vi "File Namer.vi"() -> ()   [LabVIEW 2024]
uses:
  Controls/MainStates.ctl
  <userlib>/_OpenG.lib/array/array.llb/Remove Duplicates from 1D Array (String)__ogtk.vi
  <userlib>/_OpenG.lib/array/array.llb/openg_array.lvlib
panel:
  in  "Clean after \"(\"":bool
  out "New":string
  out "Old":string
  out "new path":path
  in  "Auto":enum32{"Manual", "MKV", "AVI", "MP4", "MP3"}(radio)
  in  "Commit":bool
  in  "Replacement String":string
  in  "Split Key":string="("
  in  "Method":T1(ring)
  in  "Extension":string=".*"
  in  "Path":path
  out "New":i32(listbox)
  out "Current":i32(listbox)=1
  in  "Exit":bool
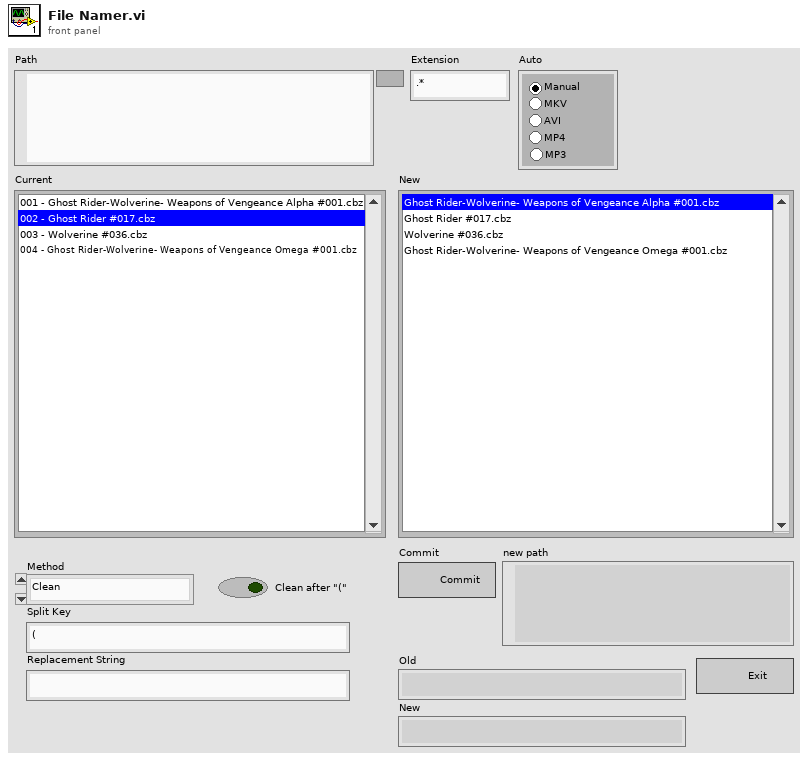
[diagram p1: front panel]
types:
  T1 = enum16{"Clean", "Replace", "Clear Periods", "Strip Prefix", "Add Prefix"}
  T2 = typedef "MainStates.ctl" = enum16{"Init", "Get Path", "Get Files", "Set Extension", "Check for Dups", "Clean", "Add Prefix", "Replace", "Periods", "Strip Prefix", "Commit", "Wait for Input", "Exit"}
  T3 = enum8{"Enabled", "Disabled", "Disabled and Grayed Out"}
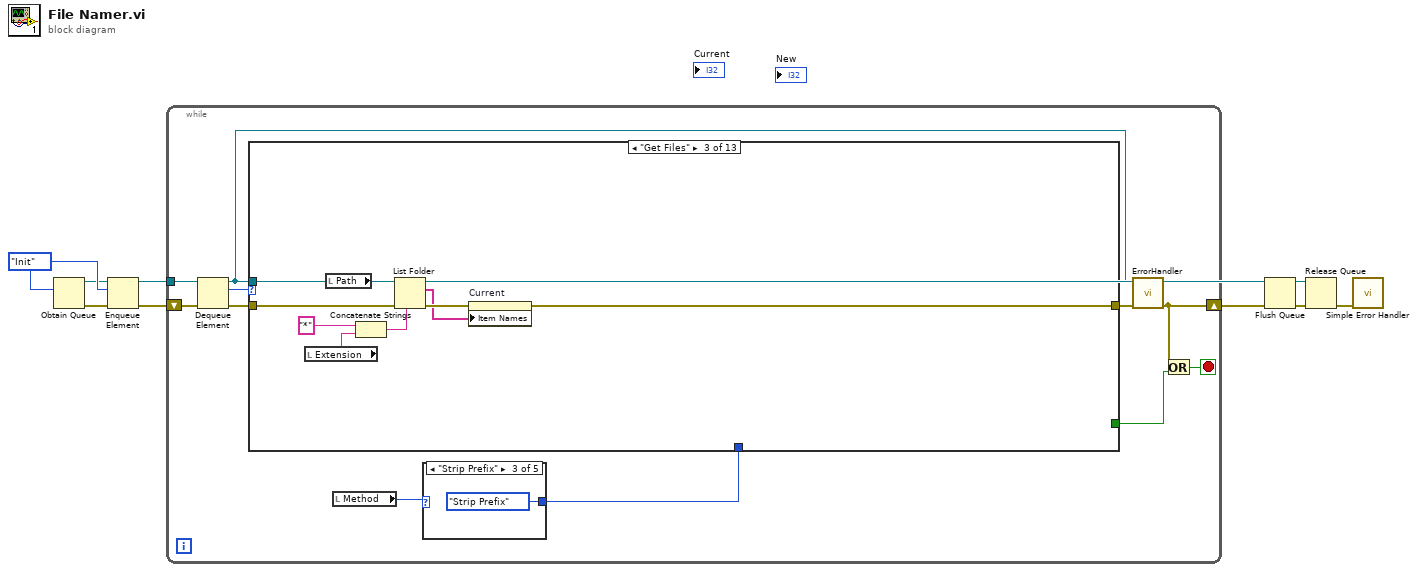
[diagram p0: block diagram]
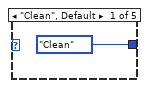
[diagram p2: hidden frame]
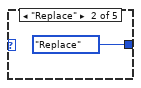
[diagram p3: hidden frame]
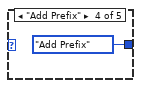
[diagram p4: hidden frame]
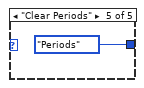
[diagram p5: hidden frame]
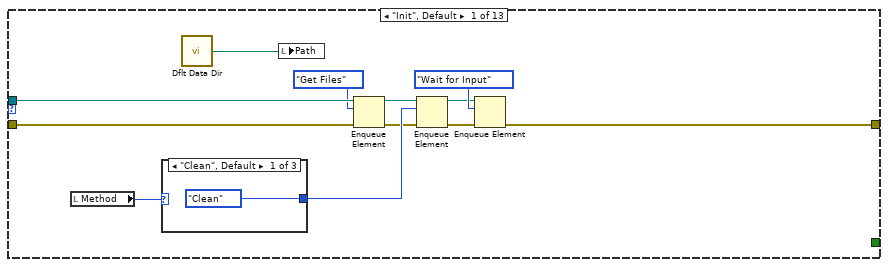
[diagram p6: hidden frame]
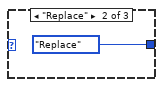
[diagram p7: hidden frame]
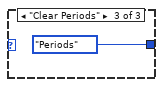
[diagram p8: hidden frame]
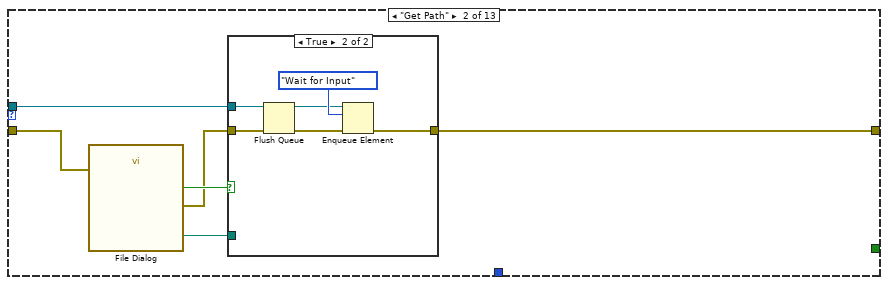
[diagram p9: hidden frame]
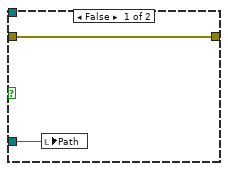
[diagram p10: hidden frame]
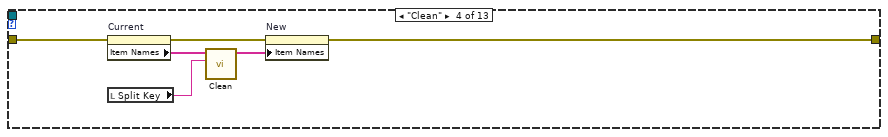
[diagram p11: hidden frame]
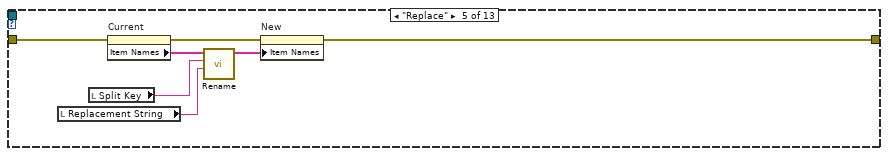
[diagram p12: hidden frame]
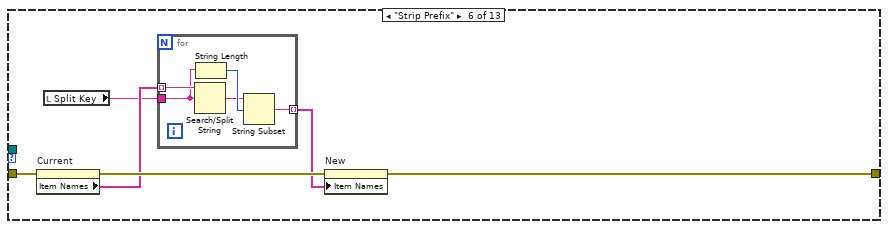
[diagram p13: hidden frame]
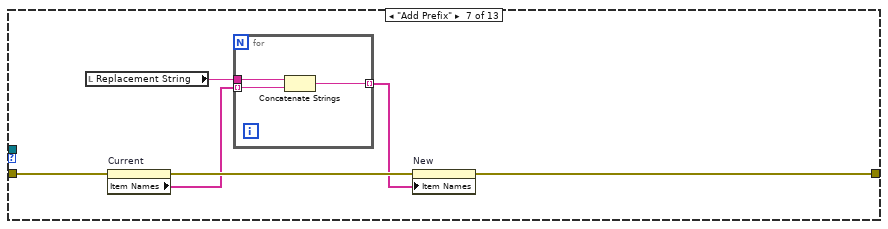
[diagram p14: hidden frame]
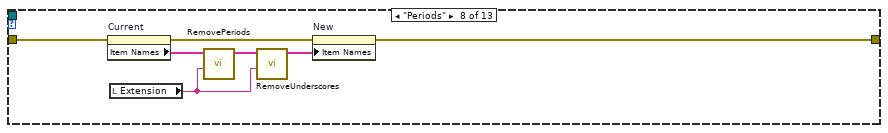
[diagram p15: hidden frame]
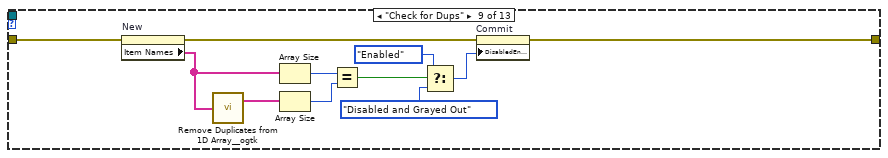
[diagram p16: hidden frame]
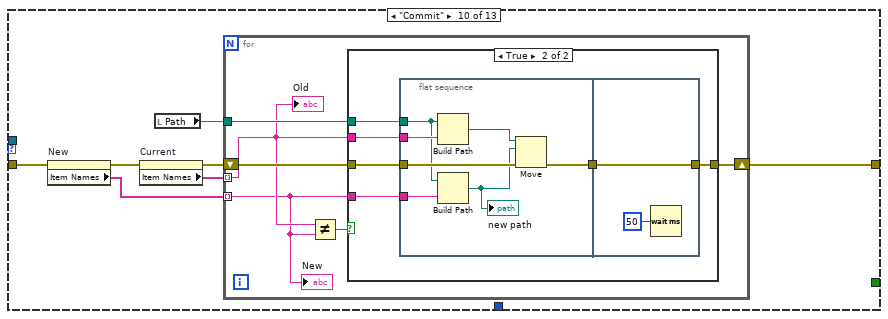
[diagram p17: hidden frame]
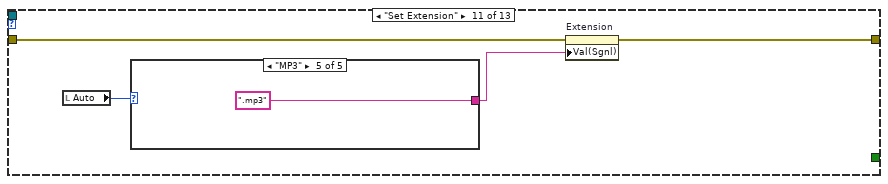
[diagram p19: hidden frame]
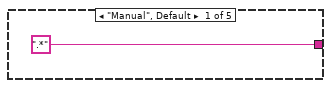
[diagram p20: hidden frame]
diagram:
  w9 = MainStates."Init" ("Main States")
  n1 = Obtain Queue(element data type=w9) -> (queue out=w8:refnum<queue>, error out=w7:errorcluster)  [unwired: 4 in, 1 out]
  n2 = Enqueue Element(queue=w8, element=w9, error in (no error)=w7) -> (queue out=w4:refnum<queue>, error out=w6:errorcluster)  [unwired: 1 in, 1 out]
  n3 = while {
    tunnel: w4 -> [w19]
    shift-right: [w11] -> w3
    shift-left: w6 -> [w20]
    stop <- w13 stop-if-true
    n4 = Dequeue Element(queue=w19, error in (no error)=w20) -> (queue out=w10:refnum<queue>, element=w18:T2, error out=w17:errorcluster)  [unwired: 1 in, 1 out]
    n5 = local read "Method"() -> (w16:T1)
    n6 = case shown="\"Strip Prefix\"" w16 {
      tunnel: [MainStates."Clean" ("Main States") MainStates."Replace" ("Main States") MainStates."Strip Prefix" ("Main States") MainStates."Add Prefix" ("Main States") MainStates."Periods" ("Main States")] -> w15
      frame "Clean", Default {
      }
      frame "Replace" {
      }
      frame "Strip Prefix" {
      }
      frame "Add Prefix" {
      }
      frame "Clear Periods" {
      }
    }
    n7 = case shown="\"Get Files\"" w18 {
      tunnel: w10 -> [w35 w44 _ _ _ _ _ _ _ _ _ w156 _]
      tunnel: w17 -> [w34 w46 w61 w68 w75 w81 w92 w102 w113 w118 w145 w155 w227]
      tunnel: [w36 w42 w55 w63 w69 w79 w90 w99 w106 w114 w143 w154 w227] -> w12
      tunnel: [_ _ _ _ _ _ _ _ _ _ _ _ TRUE] -> w14
      tunnel: w15 -> [_ _ _ _ _ _ _ _ _ _ _ w153 _]
      frame "Init", Default {
        n8 = local read "Method"() -> (w33:T1)
        n9 = case shown="\"Clean\", Default" w33 {
          tunnel: [MainStates."Clean" ("Main States") MainStates."Replace" ("Main States") MainStates."Periods" ("Main States")] -> w30
          frame "Clean", Default {
          }
          frame "Replace" {
          }
          frame "Clear Periods" {
          }
        }
        n10 = call <vilib>:"Dflt Data Dir.vi"() -> ("App:Default Data Directory"=w26:path)
        n11 = local write "Path"(w26) -> ()
        n12 = Enqueue Element(queue=w35, element=MainStates."Get Files" ("Main States"), error in (no error)=w34) -> (queue out=w28:refnum<queue>, error out=w27:errorcluster)  [unwired: 1 in, 1 out]
        n13 = Enqueue Element(queue=w28, element=w30, error in (no error)=w27) -> (queue out=w31:refnum<queue>, error out=w32:errorcluster)  [unwired: 1 in, 1 out]
        n14 = Enqueue Element(queue=w31, element=MainStates."Wait for Input" ("Main States"), error in (no error)=w32) -> (error out=w36:errorcluster)  [unwired: 1 in, 2 out]
      }
      frame "Get Path" {
        n15 = call "File Dialog"("error in"=w46) -> ("selected path"=w41:path, "cancelled"=w45:bool, "error out"=w43:errorcluster)  [unwired: 11 in, 1 out]
        n16 = case shown="True" w45 {
          tunnel: w44 -> [_ w54]
          tunnel: w43 -> [w47 w53]
          tunnel: [w47 w49] -> w42
          tunnel: w41 -> [w48 _]
          frame False {
            n17 = local write "Path"(w48) -> ()
          }
          frame True {
            n18 = Flush Queue(queue=w54, error in (no error)=w53) -> (queue out=w51:refnum<queue>, error out=w50:errorcluster)  [unwired: 1 out]
            n19 = Enqueue Element(queue=w51, element=MainStates."Wait for Input" ("Main States"), error in (no error)=w50) -> (error out=w49:errorcluster)  [unwired: 1 in, 2 out]
          }
        }
      }
      frame "Get Files" {
        n20 = local read "Extension"() -> (w56:string)
        n21 = local read "Path"() -> (w62:path)
        n22 = Concatenate Strings("*", w56) -> (w57:string)
        n23 = List Folder(path=w62, pattern=w57, error in=w61) -> (filenames=w59:string[], error out=w60:errorcluster)  [unwired: 1 in, 2 out]
        n24 = property on="Current" class="LstBox (strict)"(error in=w60, "Item Names"=w59) -> (error out=w55:errorcluster)  [unwired: 1 in, 1 out]
      }
      frame "Clean" {
        n25 = property on="Current" class="LstBox (strict)"(error in=w68) -> (error out=w64:errorcluster, "Item Names"=w67:string[])  [unwired: 1 in, 1 out]
        n26 = local read "Split Key"() -> (w66:string)
        n27 = call "Clean.vi"("Split Key"=w66, "Filenames In"=w67) -> ("Filenames Out"=w65:string[])  [unwired: 9 in]
        n28 = property on="New" class="LstBox (strict)"(error in=w64, "Item Names"=w65) -> (error out=w63:errorcluster)  [unwired: 1 in, 1 out]
      }
      frame "Replace" {
        n29 = local read "Replacement String"() -> (w72:string)
        n30 = local read "Split Key"() -> (w73:string)
        n31 = property on="Current" class="LstBox (strict)"(error in=w75) -> (error out=w70:errorcluster, "Item Names"=w74:string[])  [unwired: 1 in, 1 out]
        n32 = call "Rename.vi"("Replacement String"=w72, "Split Key"=w73, "Filenames In"=w74) -> ("Filenames Out"=w71:string[])  [unwired: 8 in]
        n33 = property on="New" class="LstBox (strict)"(error in=w70, "Item Names"=w71) -> (error out=w69:errorcluster)  [unwired: 1 in, 1 out]
      }
      frame "Strip Prefix" {
        n34 = property on="Current" class="LstBox (strict)"(error in=w81) -> (error out=w80:errorcluster, "Item Names"=w78:string[])  [unwired: 1 in, 1 out]
        n35 = local read "Split Key"() -> (w77:string)
        n36 = for {
          tunnel: w78 -> [w86] mode=indexing
          tunnel: w77 -> [w85]
          tunnel: [w82] -> w76 mode=indexing
          n37 = Search/Split String(string=w86, search string/char (-)=w85) -> (match + rest of string=w83:string)  [unwired: 1 in, 2 out]
          n38 = String Length(string=w85) -> (length=w84:i32)
          n39 = String Subset(string=w83, offset (0)=w84) -> (substring=w82:string)  [unwired: 1 in]
        }
        n40 = property on="New" class="LstBox (strict)"(error in=w80, "Item Names"=w76) -> (error out=w79:errorcluster)  [unwired: 1 in, 1 out]
      }
      frame "Add Prefix" {
        n41 = local read "Replacement String"() -> (w88:string)
        n42 = property on="Current" class="LstBox (strict)"(error in=w92) -> (error out=w91:errorcluster, "Item Names"=w89:string[])  [unwired: 1 in, 1 out]
        n43 = for {
          tunnel: w89 -> [w95] mode=indexing
          tunnel: w88 -> [w94]
          tunnel: [w93] -> w87 mode=indexing
          n44 = Concatenate Strings(w94, w95) -> (w93:string)
        }
        n45 = property on="New" class="LstBox (strict)"(error in=w91, "Item Names"=w87) -> (error out=w90:errorcluster)  [unwired: 1 in, 1 out]
      }
      frame "Periods" {
        n46 = property on="Current" class="LstBox (strict)"(error in=w102) -> (error out=w100:errorcluster, "Item Names"=w101:string[])  [unwired: 1 in, 1 out]
        n47 = local read "Extension"() -> (w96:string)
        n48 = call "RemovePeriods.vi"("Extension"=w96, "Filenames In"=w101) -> ("Filenames Out"=w98:string[])  [unwired: 9 in]
        n49 = call "RemoveUnderscores.vi"("Extension"=w96, "Filenames In"=w98) -> ("Filenames Out"=w97:string[])  [unwired: 9 in]
        n50 = property on="New" class="LstBox (strict)"(error in=w100, "Item Names"=w97) -> (error out=w99:errorcluster)  [unwired: 1 in, 1 out]
      }
      frame "Check for Dups" {
        n51 = property on="New" class="LstBox (strict)"(error in=w113) -> (error out=w107:errorcluster, "Item Names"=w112:string[])  [unwired: 1 in, 1 out]
        n52 = call-poly <userlib>:"Remove Duplicates from 1D Array__ogtk.vi"("Input Array"=w112) -> ("Output Array"=w111:string[])  [unwired: 1 out]
        n53 = Array Size(array=w112) -> (size(s)=w110:i32)
        n54 = Array Size(array=w111) -> (size(s)=w109:i32)
        n55 = Equal?(x=w110, y=w109) -> (x = y?=w108:bool)
        n56 = Select(t=T3."Enabled" ("Disabled"), s=w108, f=T3."Disabled and Grayed Out" ("Disabled")) -> (s? t:f=w103:T3)
        n57 = property on="Commit" class="Bool"(error in=w107, "DisabledEnum"=w103) -> (error out=w106:errorcluster)  [unwired: 1 in, 1 out]
      }
      frame "Commit" {
        n58 = property on="New" class="LstBox (strict)"(error in=w118) -> (error out=w117:errorcluster, "Item Names"=w116:string[])  [unwired: 1 in, 1 out]
        n59 = property on="Current" class="LstBox (strict)"(error in=w117) -> (error out=w115:errorcluster, "Item Names"=w119:string[])  [unwired: 1 in, 1 out]
        n60 = local read "Path"() -> (w120:path)
        n61 = for {
          tunnel: w120 -> [w125]
          tunnel: w119 -> [w122] mode=indexing
          tunnel: w116 -> [w121] mode=indexing
          shift-right: [w124] -> w114
          shift-left: w115 -> [w126]
          n62 = Not Equal?(x=w122, y=w121) -> (x != y?=w123:bool)
          n63 = case shown="True" w123 {
            tunnel: w122 -> [_ w133]
            tunnel: w126 -> [w127 w132]
            tunnel: w125 -> [_ w131]
            tunnel: w121 -> [_ w130]
            tunnel: [w127 w129] -> w124
            frame False {
            }
            frame True {
              n64 = flat-sequence {
                tunnel: w133 -> [w140]
                tunnel: w132 -> [w139]
                tunnel: w131 -> [w138]
                tunnel: w130 -> [w137]
                tunnel: [w134] -> w128
                tunnel: [w142] -> w129
                tunnel: w128 -> [w142]
                frame #0 {
                  n65 = Build Path(base path=w138, name or relative path=w140) -> (appended path=w136:path)
                  n66 = Build Path(base path=w138, name or relative path=w137) -> (appended path=w135:path)
                  "new path" <- w135
                  n67 = Move(source path=w136, error in=w139, 10:w135) -> (error out=w134:errorcluster)  [unwired: 2 in, 2 out]
                }
                frame #1 {
                  n68 = Wait (ms)(milliseconds to wait=u32 50) -> ()  [unwired: 1 out]
                }
              }
            }
          }
          "Old" <- w122
          "New" <- w121
        }
      }
      frame "Set Extension" {
        n69 = local read "Auto"() -> (w146:enum32{"Manual", "MKV", "AVI", "MP4", "MP3"})
        n70 = case shown="\"MP3\"" w146 {
          tunnel: [".*" ".mkv" ".avi" ".mp4" ".mp3"] -> w144
          frame "Manual", Default {
          }
          frame "MKV" {
          }
          frame "AVI" {
          }
          frame "MP4" {
          }
          frame "MP3" {
          }
        }
        n71 = property on="Extension" class="Str"(error in=w145, "Val(Sgnl)"=w144) -> (error out=w143:errorcluster)  [unwired: 1 in, 1 out]
      }
      frame "Wait for Input" {
        n72 = event shown="[1] Timeout" {
          selector: _ -> [_ _ _ _ _ _ _ _]
          dyn-events: _ -> [_ _ _ _ _ _ _ _]
          timeout: 100 -> [_ _ _ _ _ _ _ _]
          tunnel: w156 -> [w160 w172 w179 w195 w208 w216 w220 w224]
          tunnel: w155 -> [w159 w171 w180 w196 w207 w214 w219 w223]
          tunnel: [w158 w169 w174 w188 w205 w210 w221 w225] -> w154
          tunnel: w153 -> [_ w168 _ w187 w203 _ _ _]
          event "Exit": Value Change {
            n73 = event-data() -> ()  [unwired: 1 in, 1 out]
            n74 = Enqueue Element(queue=w160, element=MainStates."Exit" ("Main States"), error in (no error)=w159) -> (error out=w158:errorcluster)  [unwired: 1 in, 2 out]
          }
          event Timeout {
            n75 = event-data() -> ()  [unwired: 1 in, 3 out]
            n76 = Enqueue Element(queue=w172, element=MainStates."Get Files" ("Main States"), error in (no error)=w171) -> (queue out=w166:refnum<queue>, error out=w165:errorcluster)  [unwired: 1 in, 1 out]
            n77 = Enqueue Element(queue=w166, element=w168, error in (no error)=w165) -> (queue out=w164:refnum<queue>, error out=w163:errorcluster)  [unwired: 1 in, 1 out]
            n78 = Enqueue Element(queue=w164, element=MainStates."Check for Dups" ("Main States"), error in (no error)=w163) -> (queue out=w162:refnum<queue>, error out=w161:errorcluster)  [unwired: 1 in, 1 out]
            n79 = Enqueue Element(queue=w162, element=MainStates."Wait for Input" ("Main States"), error in (no error)=w161) -> (error out=w169:errorcluster)  [unwired: 1 in, 2 out]
          }
          event "Method", "Replacement String", "Split Key": Value Change {
            n80 = event-data() -> ()  [unwired: 1 in, 1 out]
            n81 = case shown="\"Clean\", Default" "Method" {
              tunnel: [MainStates."Clean" ("Main States") MainStates."Replace" ("Main States") MainStates."Strip Prefix" ("Main States") MainStates."Add Prefix" ("Main States") MainStates."Periods" ("Main States")] -> w178
              frame "Clean", Default {
              }
              frame "Replace" {
              }
              frame "Strip Prefix" {
              }
              frame "Add Prefix" {
              }
              frame "Clear Periods" {
              }
            }
            n82 = Enqueue Element(queue=w179, element=w178, error in (no error)=w180) -> (queue out=w175:refnum<queue>, error out=w176:errorcluster)  [unwired: 1 in, 1 out]
            n83 = Enqueue Element(queue=w175, element=MainStates."Wait for Input" ("Main States"), error in (no error)=w176) -> (error out=w174:errorcluster)  [unwired: 1 in, 2 out]
          }
          event "Extension": Value Change {
            n84 = event-data() -> ()  [unwired: 1 in, 1 out]
            n85 = Enqueue Element(queue=w195, element=MainStates."Get Files" ("Main States"), error in (no error)=w196) -> (queue out=w192:refnum<queue>, error out=w193:errorcluster)  [unwired: 1 in, 1 out]
            n86 = Enqueue Element(queue=w192, element=w187, error in (no error)=w193) -> (queue out=w190:refnum<queue>, error out=w189:errorcluster)  [unwired: 1 in, 1 out]
            n87 = Enqueue Element(queue=w190, element=MainStates."Wait for Input" ("Main States"), error in (no error)=w189) -> (error out=w188:errorcluster)  [unwired: 1 in, 2 out]
          }
          event "Commit": Value Change {
            n88 = event-data() -> ()  [unwired: 1 in, 1 out]
            n89 = Enqueue Element(queue=w208, element=MainStates."Commit" ("Main States"), error in (no error)=w207) -> (queue out=w201:refnum<queue>, error out=w202:errorcluster)  [unwired: 1 in, 1 out]
            n90 = Enqueue Element(queue=w201, element=MainStates."Get Files" ("Main States"), error in (no error)=w202) -> (queue out=w200:refnum<queue>, error out=w199:errorcluster)  [unwired: 1 in, 1 out]
            n91 = Enqueue Element(queue=w200, element=w203, error in (no error)=w199) -> (queue out=w197:refnum<queue>, error out=w198:errorcluster)  [unwired: 1 in, 1 out]
            n92 = Enqueue Element(queue=w197, element=MainStates."Wait for Input" ("Main States"), error in (no error)=w198) -> (error out=w205:errorcluster)  [unwired: 1 in, 2 out]
          }
          event "Auto": Value Change {
            n93 = event-data() -> ()  [unwired: 1 in, 1 out]
            n94 = Enqueue Element(queue=w216, element=MainStates."Set Extension" ("Main States"), error in (no error)=w214) -> (queue out=w211:refnum<queue>, error out=w212:errorcluster)  [unwired: 1 in, 1 out]
            n95 = Enqueue Element(queue=w211, element=MainStates."Wait for Input" ("Main States"), error in (no error)=w212) -> (error out=w210:errorcluster)  [unwired: 1 in, 2 out]
          }
          event "Clean after \"(\"": Value Change {
            n96 = event-data() -> ()  [unwired: 1 in, 1 out]
            n97 = property on="Split Key" class="Str"(error in=w219, "Val(Sgnl)"="(" ("Split Key")) -> (error out=w218:errorcluster)  [unwired: 1 in, 1 out]
            n98 = Enqueue Element(queue=w220, element=MainStates."Wait for Input" ("Main States"), error in (no error)=w218) -> (error out=w221:errorcluster)  [unwired: 1 in, 2 out]
          }
          event "Path": Value Change {
            n99 = event-data() -> ()  [unwired: 1 in, 1 out]
            n100 = Enqueue Element(queue=w224, element=MainStates."Wait for Input" ("Main States"), error in (no error)=w223) -> (error out=w225:errorcluster)  [unwired: 1 in, 2 out]
          }
        }
      }
      frame "Exit" {
      }
    }
    n101 = call "ErrorHandler.vi"("error in (no error)"=w12, "queue in"=w10) -> ("error out"=w11:errorcluster)  [unwired: 9 in]
    n102 = Or(x=w11, y=w14) -> (x .or. y?=w13:bool)
  }
  n103 = Flush Queue(queue=w4, error in (no error)=w3) -> (queue out=w1:refnum<queue>, error out=w5:errorcluster)  [unwired: 1 out]
  n104 = Release Queue(queue=w1, error in (no error)=w5) -> (error out=w2:errorcluster)  [unwired: 1 in, 2 out]
  n105 = call <vilib>:"Simple Error Handler.vi"("error in (no error)"=w2) -> ()  [unwired: 4 in, 5 out]
